vi "Image Processing Practice.vi"() -> ()   [LabVIEW 2016]
uses:
  <vilib>/vision/NI_Vision_Development_Module.lvlib
  Robot Global Data.vi
panel:
  out "Degrees to turn":dbl
  out "Turn Direction":string
  out "abs(x)":dbl
  out "Hook found":bool
  out "Turn left/right":bool
  out "Hook-robot":dbl
  out "Hook Center":dbl
  out "x-y":dbl
  out "Hook Found In False Case 2":bool
  out "x/y 2":dbl
  out "x/y":dbl
  out "Particle Measurements (Pixels)":dbl[][](array[numeric]) format="%.2f"
  in  "Pixel Measurements 2":T1[](array[typedef]) items=["Center of Mass X", "Center of Mass Y", "First Pixel X", "First Pixel Y", "Bounding Rect Left", "Bounding Rect Top", "Bounding Rect Right", "Bounding Rect Bottom", "Max Feret Diameter Start X", "Max Feret Diameter Start Y", "Max Feret Diameter End X", "Max Feret Diameter End Y", "Max Horiz. Segment Length Left", "Max Horiz. Segment Length Right", "Max Horiz. Segment Length Row", "-", "Bounding Rect Width", "Bounding Rect Height", "Bounding Rect Diagonal", "Perimeter", "Convex Hull Perimeter", "Holes' Perimeter", "Max Feret Diameter", "Equivalent Ellipse Major Axis", "Equivalent Ellipse Minor Axis", "Equivalent Ellipse Minor Axis (Feret)", "Equivalent Rect Long Side", "Equivalent Rect Short Side", "Equivalent Rect Diagonal", "Equivalent Rect Short Side (Feret)", "Average Horiz. Segment Length", "Average Vert. Segment Length", "Hydraulic Radius", "Waddel Disk Diameter", "-", "Area", "Holes' Area", "Particle & Holes' Area", "Convex Hull Area", "Image Area", "-", "Number of Holes", "Number of Horiz. Segments", "Number of Vert. Segments", "-", "Orientation", "Max Feret Diameter Orientation", "-", "% Area/Image Area", "% Area/(Particle & Holes' Area)", "Ratio of Equivalent Ellipse Axes", "Ratio of Equivalent Rect Sides", "-", "Elongation Factor", "Compactness Factor", "Heywood Circularity Factor", "Type Factor", "-", "Sum X", "Sum Y", "Sum XX", "Sum XY", "Sum YY", "Sum XXX", "Sum XXY", "Sum XYY", "Sum YYY", "-", "Moment of Inertia XX", "Moment of Inertia XY", "Moment of Inertia YY", "Moment of Inertia XXX", "Moment of Inertia XXY", "Moment of Inertia XYY", "Moment of Inertia YYY", "Norm. Moment of Inertia XX", "Norm. Moment of Inertia XY", "Norm. Moment of Inertia YY", "Norm. Moment of Inertia XXX", "Norm. Moment of Inertia XXY", "Norm. Moment of Inertia XYY", "Norm. Moment of Inertia YYY", "Hu Moment 1", "Hu Moment 2", "Hu Moment 3", "Hu Moment 4", "Hu Moment 5", "Hu Moment 6", "Hu Moment 7"]
  out "subarray":dbl[](array[numeric])
  out "Results 2":T2 {"Score" format="%#_3g"; "Pixels"."Rectangle"."Numeric 5" format="%#_3g"; "Pixels"."Rectangle"."Numeric 3" format="%#_3g"; "Pixels"."Rectangle"."Numeric 2" format="%#_3g"; "Pixels"."Rectangle"."Numeric" format="%#_3g"; "Normalized"."Rectangle"."Numeric 5" format="%#_2g"; "Normalized"."Rectangle"."Numeric 3" format="%#_2g"; "Normalized"."Rectangle"."Numeric 2" format="%#_2g"; "Normalized"."Rectangle"."Numeric" format="%#_2g"; "Normalized"."Center"."?" format="%#_3g"; "Normalized"."Center"."?" format="%#_3g"; "Distance (ft)" format="%#_3g"}
  out "Top Score 2":dbl
  in  "Annotate 2":bool=TRUE
  in  "Score Cutoff 2":dbl=50.0
  out "Image 6":T3(plugin-control)
  out "Sorted Data":dbl[][](array[numeric])
  out "Particles":i32
  in  "Min Area Size %":dbl
  in  "Pixel Measurements":T1[](array[typedef])=[35, 4, 5, 6, 7] items=["Center of Mass X", "Center of Mass Y", "First Pixel X", "First Pixel Y", "Bounding Rect Left", "Bounding Rect Top", "Bounding Rect Right", "Bounding Rect Bottom", "Max Feret Diameter Start X", "Max Feret Diameter Start Y", "Max Feret Diameter End X", "Max Feret Diameter End Y", "Max Horiz. Segment Length Left", "Max Horiz. Segment Length Right", "Max Horiz. Segment Length Row", "-", "Bounding Rect Width", "Bounding Rect Height", "Bounding Rect Diagonal", "Perimeter", "Convex Hull Perimeter", "Holes' Perimeter", "Max Feret Diameter", "Equivalent Ellipse Major Axis", "Equivalent Ellipse Minor Axis", "Equivalent Ellipse Minor Axis (Feret)", "Equivalent Rect Long Side", "Equivalent Rect Short Side", "Equivalent Rect Diagonal", "Equivalent Rect Short Side (Feret)", "Average Horiz. Segment Length", "Average Vert. Segment Length", "Hydraulic Radius", "Waddel Disk Diameter", "-", "Area", "Holes' Area", "Particle & Holes' Area", "Convex Hull Area", "Image Area", "-", "Number of Holes", "Number of Horiz. Segments", "Number of Vert. Segments", "-", "Orientation", "Max Feret Diameter Orientation", "-", "% Area/Image Area", "% Area/(Particle & Holes' Area)", "Ratio of Equivalent Ellipse Axes", "Ratio of Equivalent Rect Sides", "-", "Elongation Factor", "Compactness Factor", "Heywood Circularity Factor", "Type Factor", "-", "Sum X", "Sum Y", "Sum XX", "Sum XY", "Sum YY", "Sum XXX", "Sum XXY", "Sum XYY", "Sum YYY", "-", "Moment of Inertia XX", "Moment of Inertia XY", "Moment of Inertia YY", "Moment of Inertia XXX", "Moment of Inertia XXY", "Moment of Inertia XYY", "Moment of Inertia YYY", "Norm. Moment of Inertia XX", "Norm. Moment of Inertia XY", "Norm. Moment of Inertia YY", "Norm. Moment of Inertia XXX", "Norm. Moment of Inertia XXY", "Norm. Moment of Inertia XYY", "Norm. Moment of Inertia YYY", "Hu Moment 1", "Hu Moment 2", "Hu Moment 3", "Hu Moment 4", "Hu Moment 5", "Hu Moment 6", "Hu Moment 7"]
  in  "Particle Count Limit":dbl=2.0 format="%#_13g"
  out "Image 4":T3(plugin-control)
  out "error out":errorcluster
  in  "Range":cluster{"Lower value":sgl, "Upper value":sgl}={"Lower value"=128.0, "Upper value"=255.0} {"Upper value" format="%.2f"; "Lower value" format="%.2f"}
  in  "Color Plane":i32(ring)=1 items=["Red", "Green", "Blue", "Hue", "Saturation", "Luminance", "Value", "Intensity"]
  in  "Color Mode 2":u16(ring)=3 items=["RGB", "HSL", "HSV", "HSI"]
  in  "LED Color 2":T4={"Hue"={107.81818389892578, 139.81818389892578}, "Sat"={176.07142857142858, 255.0}, "Val"={40.53571428571429, 255.0}} {"Hue" scale=0.0..255.0 scale format="%#_3g"}
  in  "Color Plane 2":i32(ring)=7 items=["Red", "Green", "Blue", "Hue", "Saturation", "Luminance", "Value", "Intensity"]
  out "error out 3":errorcluster
  out "error out 2":errorcluster
  in  "error in (no error)":errorcluster
  out "Image 2":T3(plugin-control)
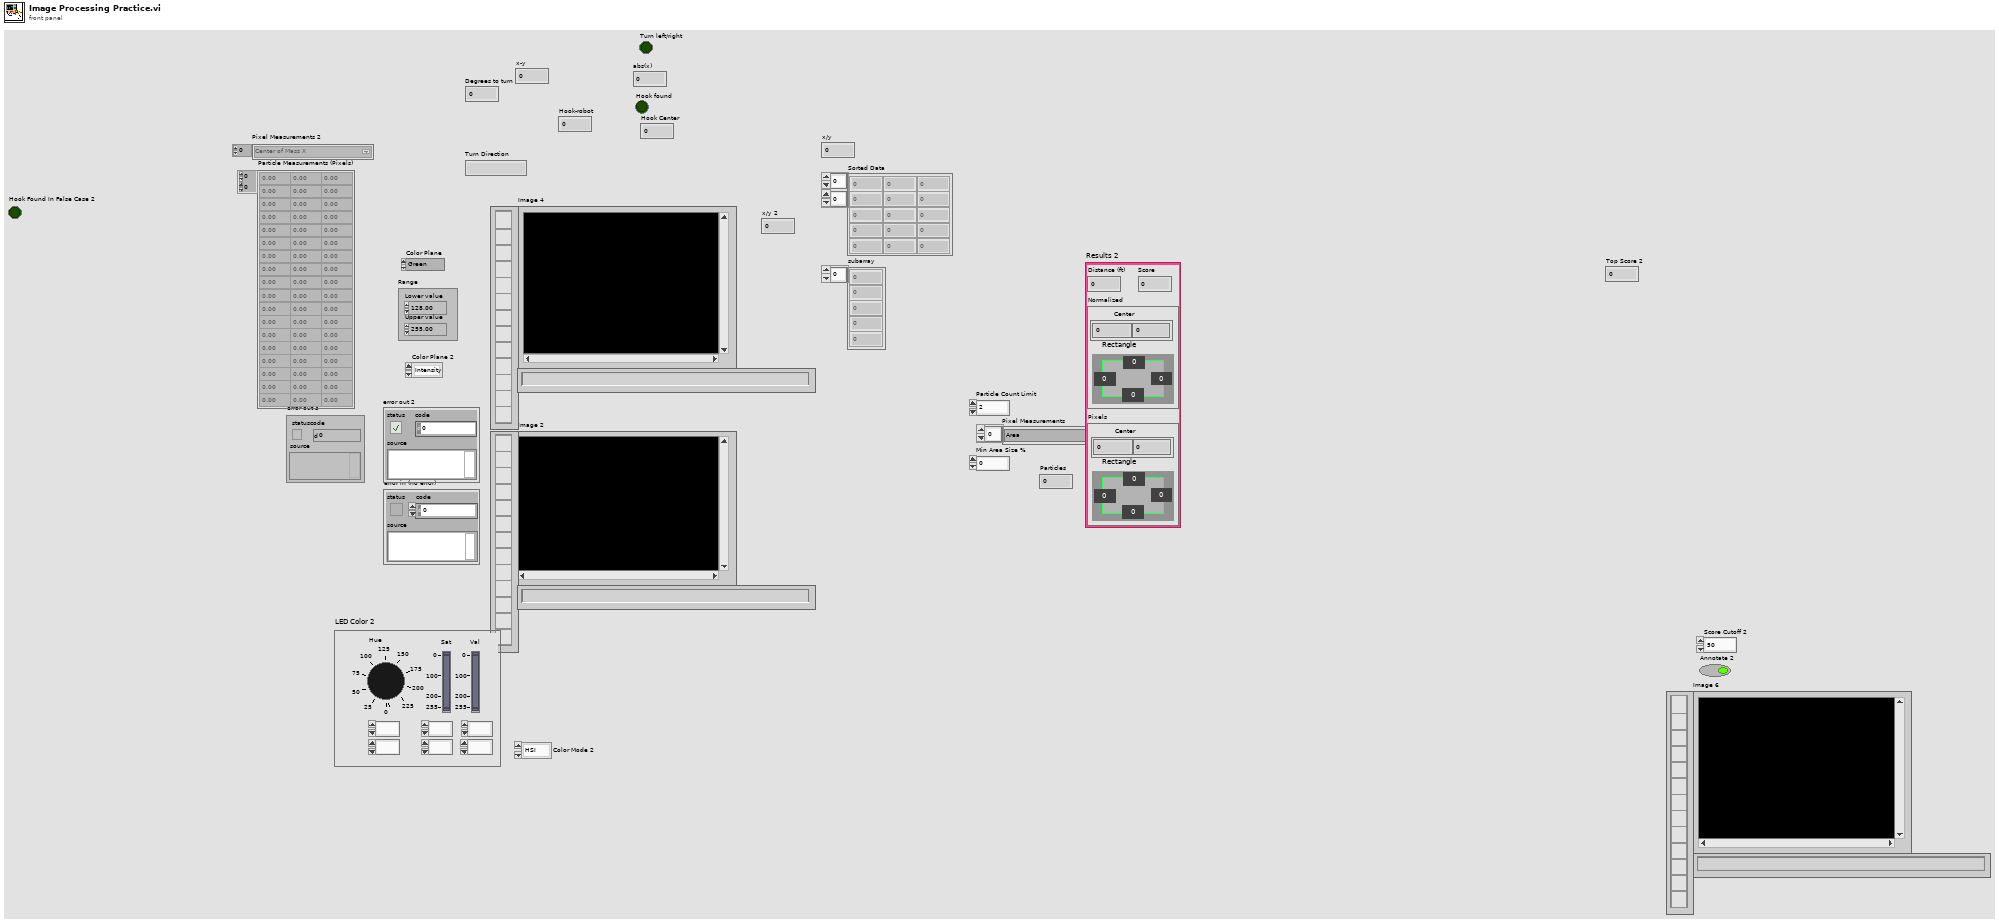
[diagram p1: front panel]
types:
  T1 = typedef "Particle Parameters" = i32
  T2 = cluster{"Distance (ft)":dbl, "Score":dbl, "Normalized":cluster{"Center":cluster{dbl, dbl}, "Rectangle":cluster{"Numeric":dbl, "Numeric 2":dbl, "Numeric 3":dbl, "Numeric 5":dbl}}, "Pixels":cluster{"Center":cluster{dbl, dbl}, "Rectangle":cluster{"Numeric":dbl, "Numeric 2":dbl, "Numeric 3":dbl, "Numeric 5":dbl}}}
  T3 = typedef "IMAQ Image.ctl" = refnum<image>
  T4 = cluster{"Hue":cluster{dbl, dbl}, "Sat":cluster{dbl, dbl}, "Val":cluster{dbl, dbl}}
  T5 = typedef "Image Type" = u32
  T6 = typedef "WPI_RobotDriveDevRef.ctl" = cluster{"DevStatus":errorcluster, "Motors[]":T7[], "Square Inputs":bool, "Max Output":dbl}
  T7 = typedef "WPI_MotorControlDeviceRef.ctl" = cluster{"DeviceStatus":errorcluster, "Type":T8, "PWM":cluster{"PWM Channel":T9, "DeadBand":T10}, "CAN":cluster{"Device Number":u8, "SetOutput VI Ref":variant, "GetOutput VI Ref":variant, "Enable VI Ref":variant, "Disable VI Ref":variant, "Data":variant}, "Invert":bool}
  T8 = typedef "WPI_MotorControlType.ctl" = enum16{"PWM", "CAN"}
  T9 = typedef "FPGA_DIOPWMChannel.ctl" = enum8{"PWM 0", "PWM 1", "PWM 2", "PWM 3", "PWM 4", "PWM 5", "PWM 6", "PWM 7", "PWM 8", "PWM 9", "PWM MXP 0", "PWM MXP 1", "PWM MXP 2", "PWM MXP 3", "PWM MXP 4", "PWM MXP 5", "PWM MXP 6", "PWM MXP 7", "PWM MXP 8", "PWM MXP 9", "Invalid"}
  T10 = typedef "WPI_PWMDeadband.ctl" = cluster{"Name":string, "maxPositivePwm":i32, "minPositivePwm":i32, "centerPwm":i32, "maxNegativePwm":i32, "minNegativePwm":i32, "angularRange":u16}
  T11 = cluster{"Left":dbl, "Top":dbl, "Right":dbl, "Bottom":dbl}
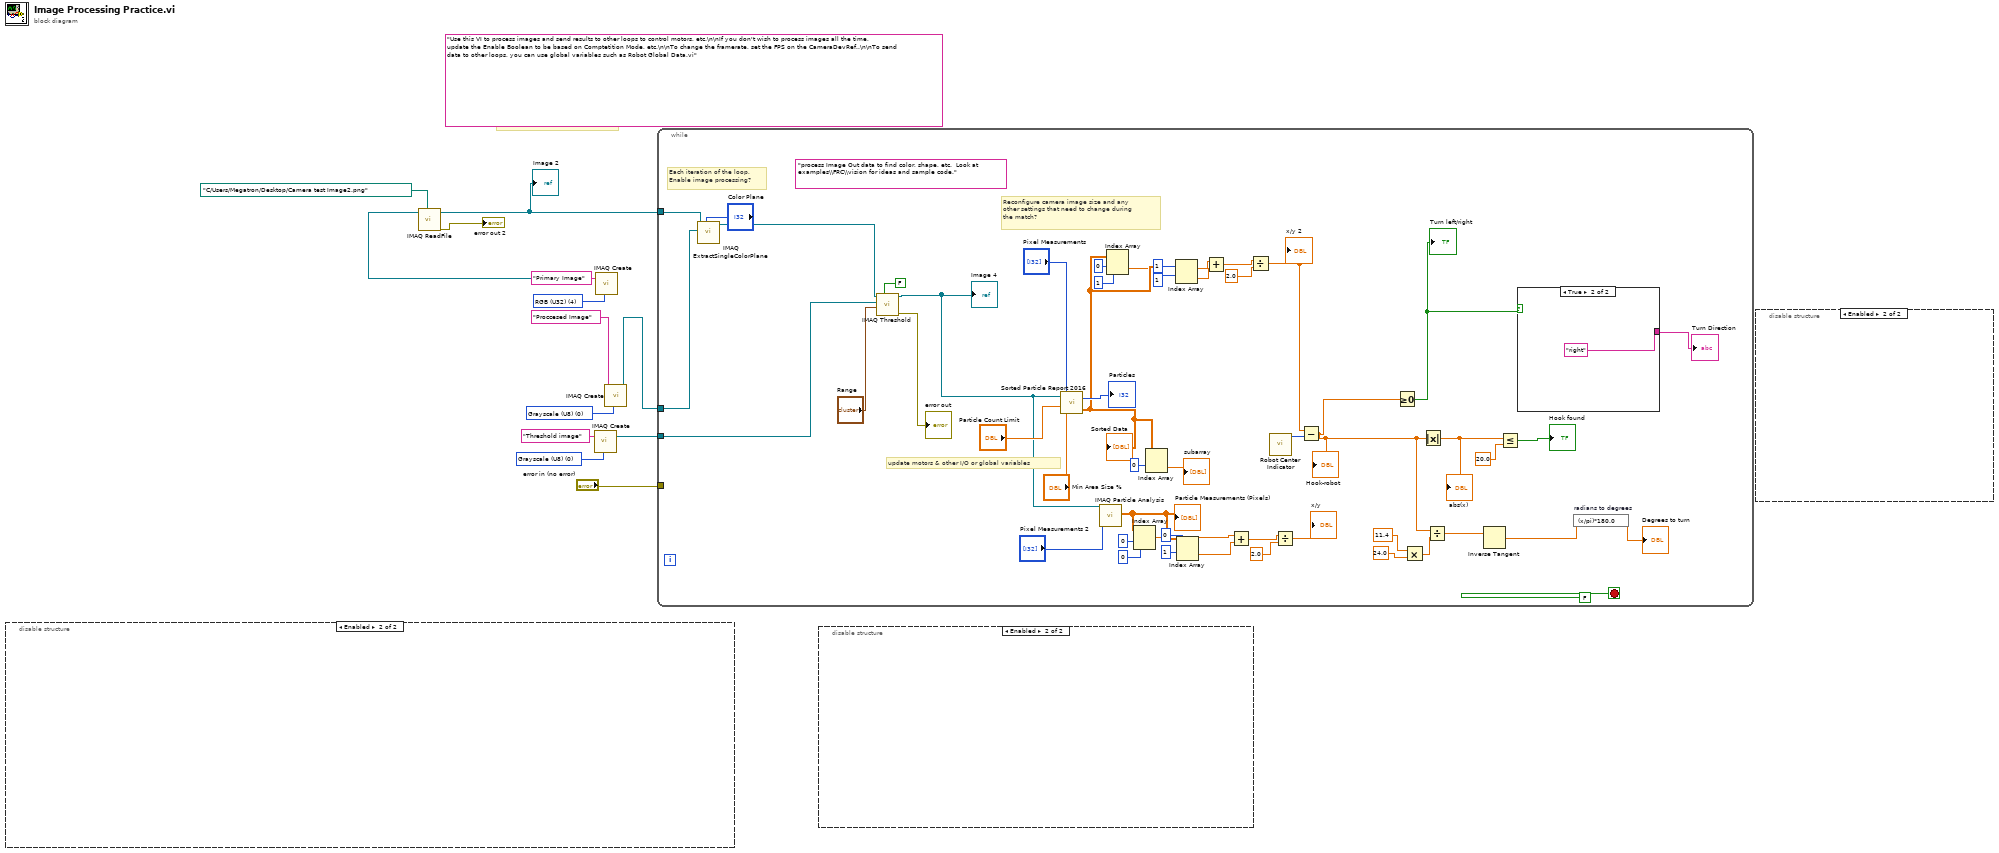
[diagram p0: block diagram]
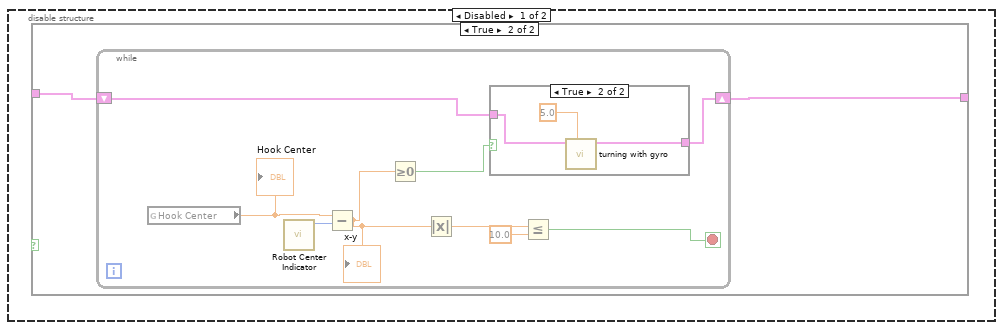
[diagram p2: hidden frame]
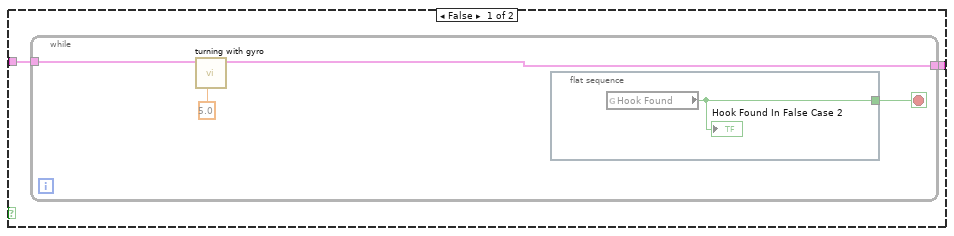
[diagram p3: hidden frame]
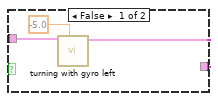
[diagram p4: hidden frame]
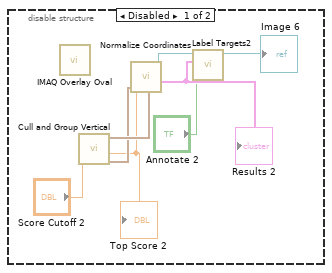
[diagram p5: hidden frame]
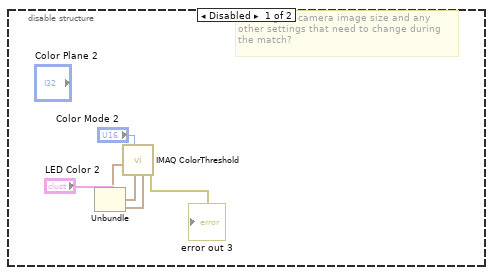
[diagram p6: hidden frame]
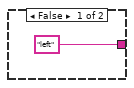
[diagram p7: hidden frame]
diagram:
  w6 = T5 0 items=["Grayscale (U8)", "Grayscale (I16)", "Grayscale (SGL)", "Complex (CSG)", "RGB (U32)", "HSL (U32)", "RGB (U64)"] ("Image Type")
  w9 = T5 0 items=["Grayscale (U8)", "Grayscale (I16)", "Grayscale (SGL)", "Complex (CSG)", "RGB (U32)", "HSL (U32)", "RGB (U64)"] ("Image Type")
  (unwired) "Use this VI to process images and send results to other loops to control motors, etc.\n\nIf you don't wish to process images all the time, update the Enable Boolean to be based on Comptetition Mode, etc.\n\nTo change the framerate, set the FPS on the CameraDevRef..\n\nTo send data to other loops, you can use global variables such as Robot Global Data.vi"
  w13 = T5 4 items=["Grayscale (U8)", "Grayscale (I16)", "Grayscale (SGL)", "Complex (CSG)", "RGB (U32)", "HSL (U32)", "RGB (U64)"] ("Image Type")
  # "For Axis cameras, this reads\nimages continuously to avoid\nlatency. For USB, it optionally\nforwards compressed images to\nthe dashboard process."
  n1 = disable-structure shown="Enabled" {
    frame Disabled {
      n2 = case shown="True" {
        selector: _ -> [_ _]
        tunnel: [w15 w22] -> _
        tunnel: _ -> [w14 w21]
        frame False {
          n3 = while {
            tunnel: [w18] -> w15
            tunnel: w14 -> [w16]
            stop <- w19 stop-if-true
            n4 = call "turning with gyro.vi"("desired angle"=5.0, "RobotDriveDevRef"=w16) -> ("RobotDriveDevRef 2"=w18:T6)  [unwired: 8 in, 1 out]
            n5 = flat-sequence {
              tunnel: [w20] -> w19
              frame #0 {
                n6 = global read "Robot Global Data.vi" "Hook Found"() -> (w20:bool)
                "Hook Found In False Case 2" <- w20
              }
            }
          }
        }
        frame True {
          n7 = while {
            shift-right: [w27] -> w22
            shift-left: w21 -> [w28]
            stop <- w23 stop-if-true
            n8 = global read "Robot Global Data.vi" "Hook Center"() -> (w30:dbl)
            "Hook Center" <- w30
            n9 = call "Robot Center Indicator.vi"() -> ("Robot Center"=w31:i32)  [unwired: 10 in, 1 out]
            n10 = Subtract(x=w30, y=w31) -> (x-y=w26:dbl)
            "x-y" <- w26
            n11 = Greater Or Equal To 0?(x=w26) -> (x >= 0?=w29:bool)
            n12 = Absolute Value(x=w26) -> (abs(x)=w25:dbl)
            n13 = case shown="True" w29 {
              tunnel: w28 -> [w34 w37]
              tunnel: [w33 w36] -> w27
              frame False {
                n14 = call "turning with gyro left.vi"("desired angle"=-5.0, "RobotDriveDevRef"=w34) -> ("RobotDriveDevRef 2"=w33:T6)  [unwired: 8 in, 1 out]
              }
              frame True {
                n15 = call "turning with gyro.vi"("desired angle"=5.0, "RobotDriveDevRef"=w37) -> ("RobotDriveDevRef 2"=w36:T6)  [unwired: 8 in, 1 out]
              }
            }
            n16 = Less Or Equal?(x=w25, y=10.0) -> (x <= y?=w23:bool)
          }
        }
      }
    }
    frame Enabled {
    }
  }
  n17 = call "IMAQ Create"("Image Name"="Threshold image", "Image Type"=w6) -> ("New Image"=w5:T3)  [unwired: 2 in, 2 out]
  n18 = call "IMAQ Create"("Image Name"="Primary Image", "Image Type"=w13) -> ("New Image"=w3:T3)  [unwired: 2 in, 2 out]
  n19 = call "IMAQ ReadFile"("File Path"=path "C:/Users/Megatron/Desktop/Camera test Image2.png", "Image"=w3) -> ("error out"=→"error out 2":errorcluster, "Image Out"=w1:T3)  [unwired: 5 in, 3 out]
  "Image 2" <- w1
  n20 = call "IMAQ Create"("Image Name"="Proccesed Image", "Image Type"=w9) -> ("New Image"=w8:T3)  [unwired: 2 in, 2 out]
  n21 = while {
    tunnel: "error in (no error)" -> [_]
    tunnel: w8 -> [w86]
    tunnel: w5 -> [w83]
    tunnel: w1 -> [w61]
    stop <- FALSE stop-if-true
    (unwired) "process Image Out data to find color, shape, etc.  Look at examples\\FRC\\vision for ideas and sample code."
    # "update motors & other I/O or global variables"
    # "Reconfigure camera image size and any\nother settings that need to change during\nthe match?"
    # "Each iteration of the loop,\nEnable image processing?"
    n22 = call "IMAQ ExtractSingleColorPlane"("Color Plane"="Color Plane", "Image Dst"=w86, "Image Src"=w61) -> ("Image Dst Out"=w84:T3)  [unwired: 7 in, 1 out]
    n23 = call "IMAQ Threshold"("Keep/Replace Value (Replace)"=FALSE, "Range"="Range", "Image Dst"=w83, "Image Src"=w84) -> ("error out"=→"error out":errorcluster, "Image Dst Out"=w73:T3)  [unwired: 6 in]
    "Image 4" <- w73
    n24 = call "Sorted Particle Report 2016.vi"("Min Area Size %"="Min Area Size %", "Particle Count Limit"="Particle Count Limit", "Pixel Measurements"="Pixel Measurements", "Image in"=w73) -> ("Sorted Data"=w57:dbl[][], "Particles"=→"Particles":i32)
    "Sorted Data" <- w57
    n25 = call "IMAQ Particle Analysis"("Pixel Measurements"="Pixel Measurements 2", "Image"=w73) -> ("Particle Measurements (Pixels)"=w70:dbl[][])  [unwired: 3 in, 6 out]
    "Particle Measurements (Pixels)" <- w70
    n26 = Index Array(array=w57, index (row)=0, index (col)=1 ("disabled index (col)")) -> (element=w55:dbl)
    n27 = Index Array(array=w70, index (row)=0, index (col)=0 ("disabled index (col)")) -> (element=w68:dbl)
    n28 = Index Array(array=w57, index (row)=0) -> (element=→"subarray":dbl[])  [unwired: 1 in]
    n29 = Index Array(array=w57, index (row)=1, index (col)=1 ("disabled index (col)")) -> (element=w56:dbl)
    n30 = Index Array(array=w70, index (row)=1, index (col)=0 ("disabled index (col)")) -> (element=w67:dbl)
    n31 = Add(x=w55, y=w56) -> (x+y=w59:dbl)
    n32 = Add(x=w68, y=w67) -> (x+y=w66:dbl)
    n33 = Divide(x=w59, y=2.0) -> (x/y=w48:dbl)
    "x/y 2" <- w48
    n34 = call "Robot Center Indicator.vi"() -> ("Robot Center"=w51:i32)  [unwired: 10 in, 1 out]
    n35 = Divide(x=w66, y=2.0) -> (x/y=→"x/y":dbl)
    n36 = Subtract(x=w48, y=w51) -> (x-y=w44:dbl)
    "Hook-robot" <- w44
    n37 = Greater Or Equal To 0?(x=w44) -> (x >= 0?=w46:bool)
    "Turn left/right" <- w46
    n38 = Multiply(x=11.4, y=24.0) -> (x*y=w41:dbl)
    n39 = Absolute Value(x=w44) -> (abs(x)=w50:dbl)
    "abs(x)" <- w50
    n40 = Divide(x=w44, y=w41) -> (x/y=w40:dbl)
    n41 = Inverse Tangent(1:w40) -> (0:w39:dbl)
    n42 = Less Or Equal?(x=w50, y=20.0) -> (x <= y?=→"Hook found":bool)
    n43 = case shown="True" w46 {
      tunnel: ["left" ("Turn Direction") "right" ("Turn Direction")] -> w45
      frame False {
      }
      frame True {
      }
    }
    "Turn Direction" <- w45
    n44 = expression code="(x/pi)*180.0" "radians to degrees"(w39) -> (→"Degrees to turn":dbl)
  }
  n45 = disable-structure shown="Enabled" {
    frame Disabled {
      # "Reconfigure camera image size and any\nother settings that need to change during\nthe match?"
      n46 = Unbundle("LED Color 2") -> ("Hue"=w92:cluster{dbl, dbl}, "Sat"=w93:cluster{dbl, dbl}, "Val"=w94:cluster{dbl, dbl})
      n47 = call "IMAQ ColorThreshold"("Blue or Luma or Val or Inten Range"=w94, "Green or Sat Range"=w93, "Color Mode"="Color Mode 2", "Red or Hue Range"=w92) -> ("error out"=→"error out 3":errorcluster, "Image Dst Out"=w91:T3)  [unwired: 6 in]
    }
    frame Enabled {
    }
  }
  n48 = disable-structure shown="Enabled" {
    frame Disabled {
      n49 = call "IMAQ Overlay Oval"() -> ()  [unwired: 10 in, 2 out]
      n50 = call "Cull and Group Vertical.vi"("Score Cutoff"="Score Cutoff 2") -> ("Rect"=w103:T11, "Top Score"=w102:dbl, "Center"=w104:cluster{"X":dbl, "Y":dbl})  [unwired: 8 in]
      "Top Score 2" <- w102
      n51 = call "Normalize Coordinates.vi"("Center"=w104, "Distance"=w102, "Bounding box"=w103) -> ("Results"=w100:T2, "Image out"=w101:T3)  [unwired: 7 in]
      "Results 2" <- w100
      n52 = call "Label Targets2.vi"("Annotate"="Annotate 2", "Results"=w100, "Image in"=w101) -> ("Image out"=→"Image 6":T3)  [unwired: 8 in]
    }
    frame Enabled {
    }
  }
